vi "TextDiff.vi"(8 "error in (no error)":errorcluster, 9 "Output Folders":T5, 10 "VI 2 Screenshots in":T1, 11 "VI 1 Screenshots in":T1) -> (0 "error out":errorcluster, 2 "Description":string, 3 "appended path":path)   [LabVIEW 2015, in "VIDiff_Screenshots.lvlib"]
uses:
  Screenshots/VIDiff_Screenshots.lvlib
  Utilities/Output Folders.ctl
  Screenshots/VI Screenshots.ctl
  Screenshots/Screenshot Info.ctl
  Screenshots/Screenshot Type.ctl
  Utilities/FilePaths.ctl
  Utilities/VIDiff_Utilities.lvlib
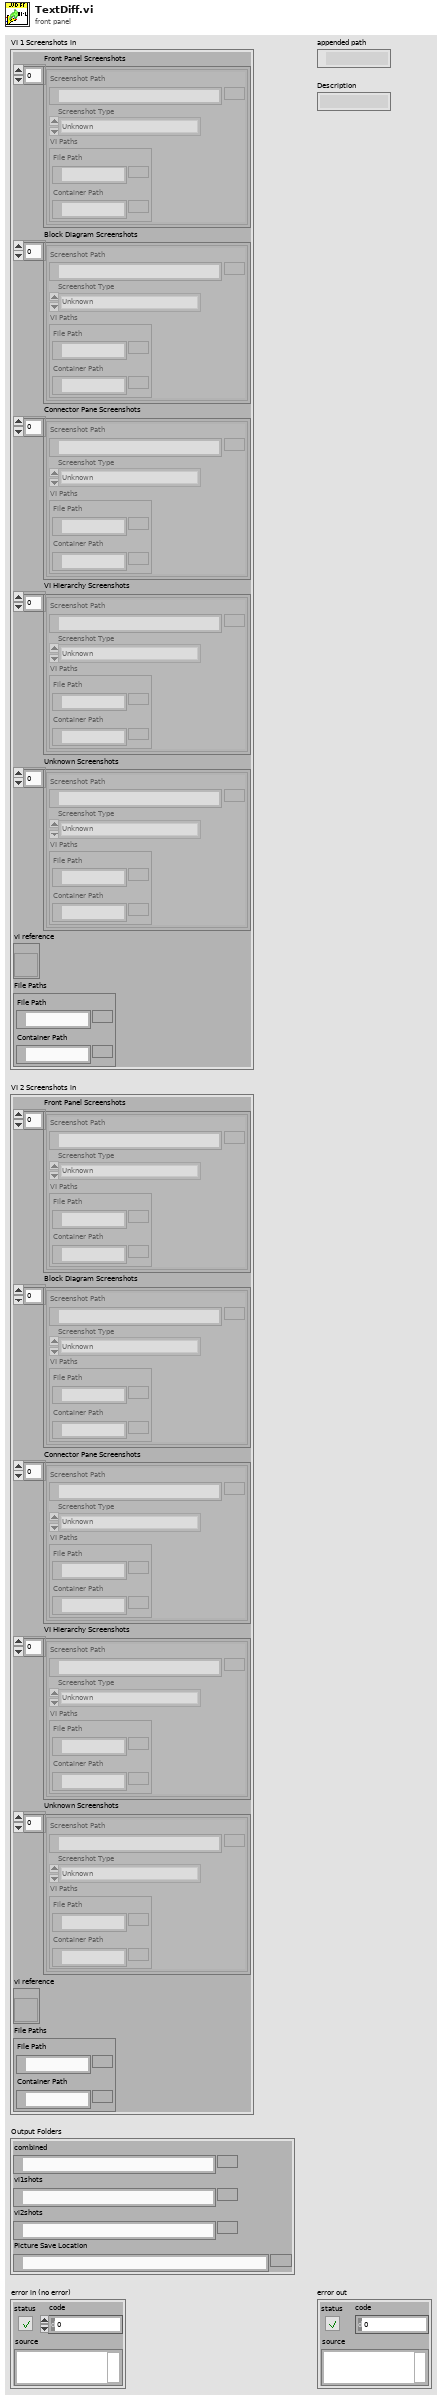
[diagram p1: front panel]
types:
  T1 = typedef "VIDiff_Screenshots.lvlib/VI Screenshots.ctl" = cluster{"Front Panel Screenshots":T2[], "Block Diagram Screenshots":T2[], "Connector Pane Screenshots":T2[], "VI Hierarchy Screenshots":T2[], "Unknown Screenshots":T2[], "vi reference":refnum<vi>, "File Paths":cluster{"File Path":path, "Container Path":path}}
  T2 = typedef "VIDiff_Screenshots.lvlib/Screenshot Info.ctl" = cluster{"Screenshot Path":path, "Screenshot Type":T3, "VI Paths":T4}
  T3 = typedef "VIDiff_Screenshots.lvlib/Screenshot Type.ctl" = enum16{"Unknown", "Front Panel", "Connector Pane", "Block Diagram", "VI Hierarchy"}
  T4 = typedef "VIDiff_Utilities.lvlib/FilePaths.ctl" = cluster{"File Path":path, "Container Path":path}
  T5 = typedef "VIDiff_Utilities.lvlib/Output Folders.ctl" = cluster{"combined":path, "vi1shots":path, "vi2shots":path, "Picture Save Location":path}
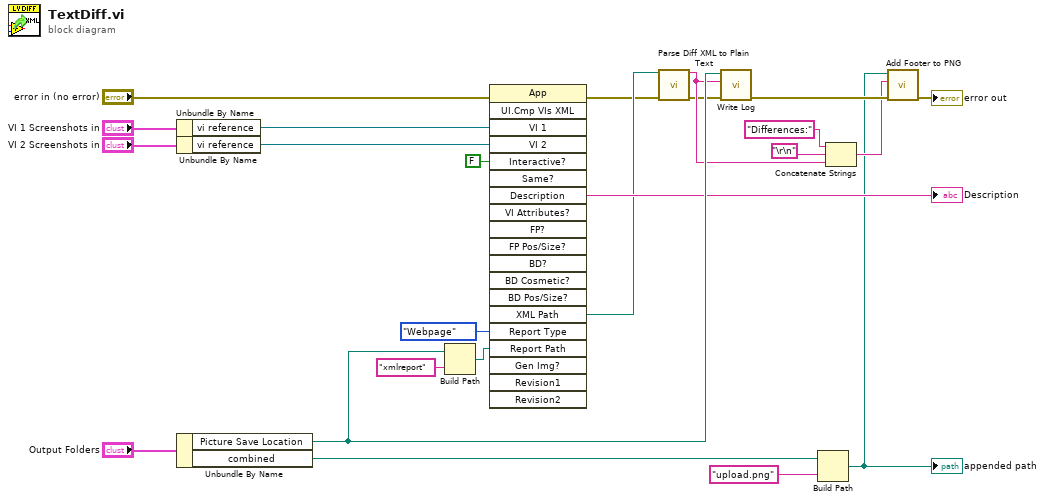
[diagram p0: block diagram]
diagram:
  n1 = Unbundle By Name("VI 1 Screenshots in") -> ("vi reference"=w20:refnum<vi>)
  n2 = Unbundle By Name("VI 2 Screenshots in") -> ("vi reference"=w21:refnum<vi>)
  n3 = Unbundle By Name("Output Folders") -> ("Picture Save Location"=w23:path, "combined"=w24:path)
  n4 = Build Path(base path=w23, name or relative path="xmlreport") -> (appended path=w14:path)
  n5 = invoke class="App" method="UI.Cmp VIs XML"(error in="error in (no error)", "VI 1"=w20, "VI 2"=w21, "Interactive?"=FALSE, "Report Type"=enum32{"None", "Webpage", "Text", "MS Word"}."Webpage", "Report Path"=w14) -> (error out=w7:errorcluster, "Description"=→"Description":string, "XML Path"=w15:path)  [unwired: 14 in, 17 out]
  n6 = call "Parse Diff XML to Plain Text.vi"("XML Path"=w15, "error in"=w7) -> ("change description"=w10:string, "error out"=w8:errorcluster)  [unwired: 12 in]
  n7 = call "Write Log.vi"("error in (no error)"=w8, "Log"=w10, "Log Folder"=w23) -> ("error out"=w9:errorcluster)  [unwired: 8 in]
  n8 = Build Path(base path=w24, name or relative path="upload.png") -> (appended path=w2:path)
  "appended path" <- w2
  n9 = Concatenate Strings("Differences:" ("string"), "\r\n", w10) -> (w5:string)
  n10 = call "Add Footer to PNG.vi"("error in (no error)"=w9, "Footer String"=w5, "PNG File"=w2) -> ("error out"=→"error out":errorcluster)  [unwired: 8 in]
